vi "Get State Transition User Event.vi"(8 "error in (no error)":errorcluster, 10 "State Transition Event Notifier":refnum<notifier>, 11 "State Actor in":refnum<class "State Actor.lvclass">) -> (0 "error out":errorcluster, 3 "State Actor out":refnum<class "State Actor.lvclass">)   [LabVIEW 2024, in "State Actor.lvlib" / "State Actor.lvclass"]
uses:
  State Actor.lvclass
  State Actor.lvclass/State Actor.ctl
  State Transition Event.ctl
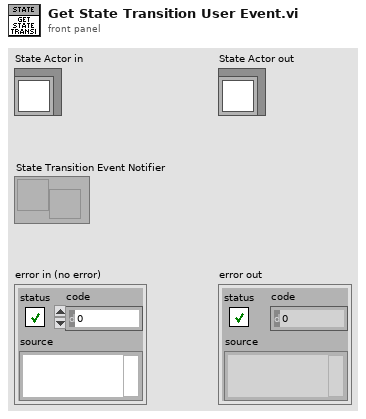
[diagram p1: front panel]
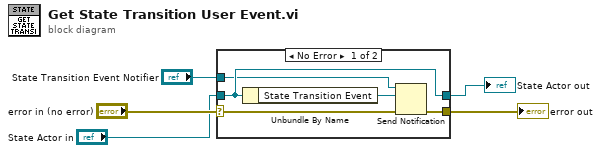
[diagram p0: block diagram]
diagram:
  n1 = case shown="No Error" "error in (no error)" {
    selector: "error in (no error)" -> [w9 w12]
    tunnel: [w8 w12] -> w4
    tunnel: [w10 w11] -> w2
    tunnel: "State Actor in" -> [w10 w11]
    tunnel: "State Transition Event Notifier" -> [w7 _]
    frame No Error {
      n2 = Unbundle By Name(w10) -> ("State Transition Event"=w6:refnum<user-event>)
      n3 = Send Notification(notification=w6, notifier=w7, error in (no error)=w9) -> (error out=w8:errorcluster)  [unwired: 1 out]
    }
    frame Error {
    }
  }
  "error out" <- w4
  "State Actor out" <- w2
